vi "单向扫描.vi"(5 "电压改变量":dbl, 7 "极限电流(mA)":dbl, 8 "错误输入":errorcluster, 10 "扫描电压(V)":dbl, 11 "VISA资源名称":refnum<visa-resource-name>) -> (0 "错误输出":errorcluster, 1 "时间标识":timestamp, 2 "扫描数据":dbl[][](array[numeric]), 3 "VISA资源名称输出":refnum<visa-resource-name>)   [LabVIEW 2019]
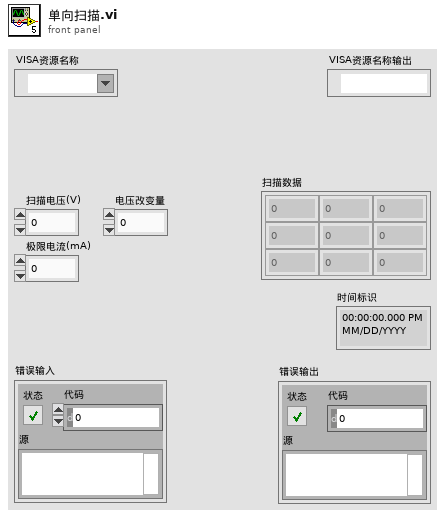
[diagram p1: front panel]
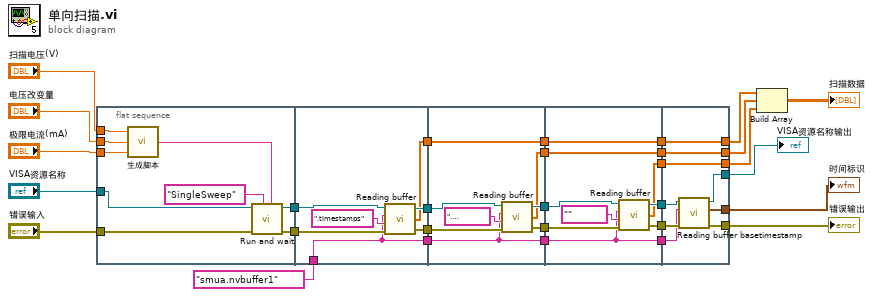
[diagram p0: block diagram]
diagram:
  n1 = flat-sequence {
    tunnel: "扫描电压(V)" -> [w38]
    tunnel: "电压改变量" -> [w35]
    tunnel: "极限电流(mA)" -> [w37]
    tunnel: "错误输入" -> [w34]
    tunnel: "VISA资源名称" -> [w33]
    tunnel: [w32] -> w25
    tunnel: [w31] -> w24
    tunnel: w25 -> [w45]
    tunnel: w24 -> [w44]
    tunnel: [w43] -> w23
    tunnel: [w42] -> w22
    tunnel: [w41] -> w14
    tunnel: "smua.nvbuffer1" ("缓冲区名称") -> [w41]
    tunnel: [w40] -> w9
    tunnel: w23 -> [w53]
    tunnel: w22 -> [w52]
    tunnel: [w51] -> w21
    tunnel: [w50] -> w20
    tunnel: w14 -> [w49]
    tunnel: [w49] -> w13
    tunnel: w9 -> [w48]
    tunnel: [w48] -> w8
    tunnel: [w47] -> w5
    tunnel: w21 -> [w62]
    tunnel: w20 -> [w61]
    tunnel: [w60] -> w16
    tunnel: [w59] -> w15
    tunnel: w13 -> [w58]
    tunnel: [w58] -> w12
    tunnel: w8 -> [w57]
    tunnel: [w57] -> w6
    tunnel: w5 -> [w56]
    tunnel: [w56] -> w4
    tunnel: [w55] -> w2
    tunnel: [w70] -> w18
    tunnel: [w69] -> w19
    tunnel: w16 -> [w72]
    tunnel: w15 -> [w71]
    tunnel: w12 -> [w68]
    tunnel: [w67] -> w11
    tunnel: [w66] -> w7
    tunnel: w6 -> [w66]
    tunnel: w4 -> [w65]
    tunnel: [w65] -> w3
    tunnel: w2 -> [w64]
    tunnel: [w64] -> w1
    frame #0 {
      n2 = call-poly "生成脚本.vi"("扫描电压(V)"=w38, "电压改变量"=w35, "极限电流(mA)"=w37) -> ("Script"=w36:string)  [unwired: 6 in]
      n3 = call "Run and wait.vi"("Script"=w36, "Script Name"="SingleSweep", "错误输入"=w34, "VISA资源名称"=w33) -> ("错误输出"=w32:errorcluster, "VISA资源名称输出"=w31:refnum<visa-resource-name>)  [unwired: 6 in]
    }
    frame #1 {
      n4 = call "Reading buffer.vi"("错误输入"=w45, "Options"=".timestamps", "缓冲区名称"=w41, "VISA资源名称"=w44) -> ("错误输出"=w42:errorcluster, "缓冲区数据"=w40:dbl[], "VISA资源名称输出"=w43:refnum<visa-resource-name>)
    }
    frame #2 {
      n5 = call "Reading buffer.vi"("错误输入"=w52, "Options"=".sourcevalues", "缓冲区名称"=w49, "VISA资源名称"=w53) -> ("错误输出"=w51:errorcluster, "缓冲区数据"=w47:dbl[], "VISA资源名称输出"=w50:refnum<visa-resource-name>)
    }
    frame #3 {
      n6 = call "Reading buffer.vi"("错误输入"=w62, "Options"="", "缓冲区名称"=w58, "VISA资源名称"=w61) -> ("错误输出"=w59:errorcluster, "缓冲区数据"=w55:dbl[], "VISA资源名称输出"=w60:refnum<visa-resource-name>)
    }
    frame #4 {
      n7 = call "Reading buffer basetimestamp.vi"("错误输入"=w71, "缓冲区名称"=w68, "VISA资源名称"=w72) -> ("错误输出"=w70:errorcluster, "时间标识"=w67:timestamp, "VISA资源名称输出"=w69:refnum<visa-resource-name>)  [unwired: 6 in]
    }
  }
  n8 = Build Array(w7, w3, w1) -> (→"扫描数据":dbl[][])
  "VISA资源名称输出" <- w19
  "错误输出" <- w18
  "时间标识" <- w11
